vi "All Child Values.vi"(11 "NewEntityTemplate in":refnum<class "MoarDemo.lvclass">) -> (2 "All Values":refnum<class "Type.lvclass">[](array[class]))   [LabVIEW 2020, in "tests.lvlib" / "MoarDemo.lvclass"]
uses:
  MoarDemo.lvclass
  <vilib>/IlluminatedG/IG Conditum Base/Conditum/Columns/Type/Type.lvclass
  MoarDemo.lvclass/MoarDemo.ctl
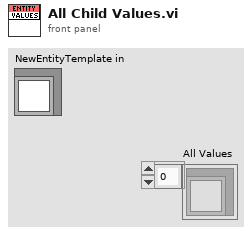
[diagram p1: front panel]
types:
  T1 = typedef "tests.lvlib/MoarDemo.lvclass/Columns.ctl" = cluster{"Active":refnum<class "Boolean.lvclass">, "Score":refnum<class "Double.lvclass">, "Name":refnum<class "String.lvclass">}
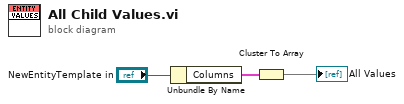
[diagram p0: block diagram]
diagram:
  n1 = Unbundle By Name("NewEntityTemplate in") -> ("Columns"=w2:T1)
  n2 = Cluster To Array(cluster=w2) -> (array=→"All Values":refnum<class "Type.lvclass">[])
